vi "Get Terminal Refs for Variant To Data.vi"(8 "error in (no error)":errorcluster, 10 "Reference in":refnum<vi>, 11 "Setter Generator In":refnum<class "Setter Generator.lvclass">) -> (0 "error out":errorcluster, 2 "reference out":refnum<vi>, 3 "Setter Generator Out":refnum<class "Setter Generator.lvclass">)   [LabVIEW 2020, in "Method Generation.lvlib" / "Setter Generator.lvclass"]
uses:
  Setter Generator.lvclass
  Setter Generator.lvclass/Setter Generator.ctl
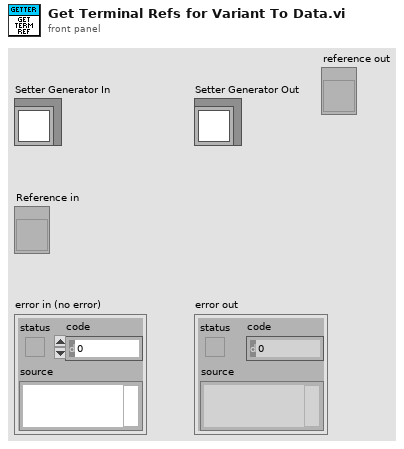
[diagram p1: front panel]
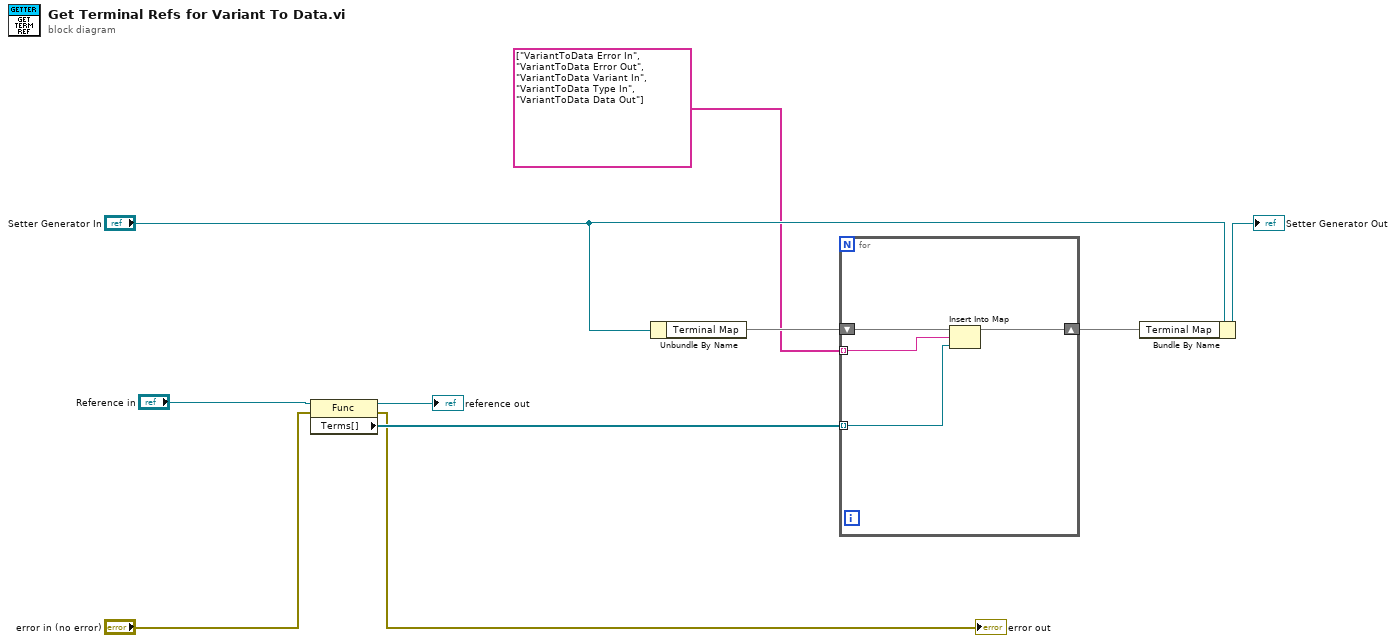
[diagram p0: block diagram]
diagram:
  n1 = property class="Func"(reference="Reference in", error in="error in (no error)") -> (reference out=→"reference out":refnum<vi>, error out=→"error out":errorcluster, "Terms[]"=w9:refnum<vi>[])
  n2 = Unbundle By Name("Setter Generator In") -> ("Terminal Map"=w6:map{string, refnum<vi>})
  n3 = for {
    tunnel: w9 -> [w11] mode=indexing
    tunnel: string[] ["VariantToData Error In", "VariantToData Error Out", "VariantToData Variant In", "VariantToData Type In", "VariantToData Data Out"] -> [w13] mode=indexing
    shift-right: [w12] -> w5
    shift-left: w6 -> [w14]
    n4 = Insert Into Map(map in=w14, key=w13, value=w11) -> (map out=w12:map{string, refnum<vi>})  [unwired: 2 out]
  }
  n5 = Bundle By Name(cluster="Setter Generator In", "Terminal Map"=w5) -> (→"Setter Generator Out":refnum<class "Setter Generator.lvclass">)
